vi "Forwards gradients.vi"(1 "Identification errors, e":dbl[][](array[numeric]) format="%.3f", 2 "Wavenet-IIR, Y":dbl[][](array[numeric]) format="%.3f", 3 "Persistent signal":dbl=1.0 min=1.0 max=10.0 step=1.0 format="%.3f") -> (0 "Forwards, D":dbl[][](array[numeric]) format="%.3f")   [LabVIEW 2022 SP3]
uses:
  <vilib>/Analysis/NI_AALBase.lvlib
  <vilib>/Analysis/baseanly.llb/Real A x B.vi
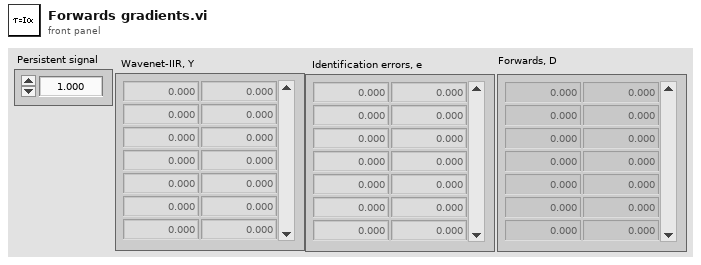
[diagram p1: front panel]
types:
  T1 = typedef "NI_Matrix.lvlib/RealMatrix.ctl" = dbl[][]
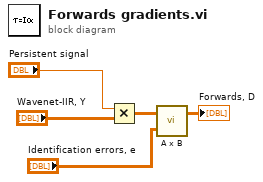
[diagram p0: block diagram]
diagram:
  n1 = Multiply(x="Persistent signal", y="Wavenet-IIR, Y") -> (x*y=w3:dbl[][])
  n2 = call-poly <vilib>:"A x B.vi"("B"="Identification errors, e", "A"=w3) -> ("A x B"=→"Forwards, D":T1)  [unwired: 1 out]
